vi "Eliminar ceros dentro de while o for V 2011.vi"() -> ()   [LabVIEW 2011]
panel:
  out "ELEMENTOS A UTILIZAR 0001  H":dbl[](array[numeric])
  out "reversed array 2":dbl[](array[numeric])
  out "reversed array":dbl[](array[numeric])
  out "appended array":dbl[](array[numeric])
  in  "stop":bool
  out "element":dbl
  in  "array":dbl[](array[numeric])=[3.0, 4.0, 0.0, 0.0, 2.0, 35.0, 0.0, 32.0, 0.0, 0.0, 12.0, 8.0, 6.0, 0.0, 2.0]
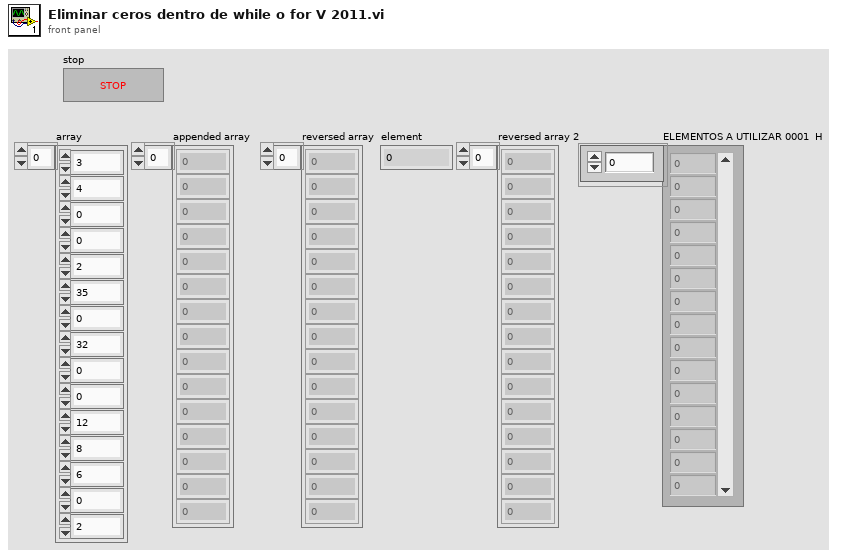
[diagram p1: front panel]
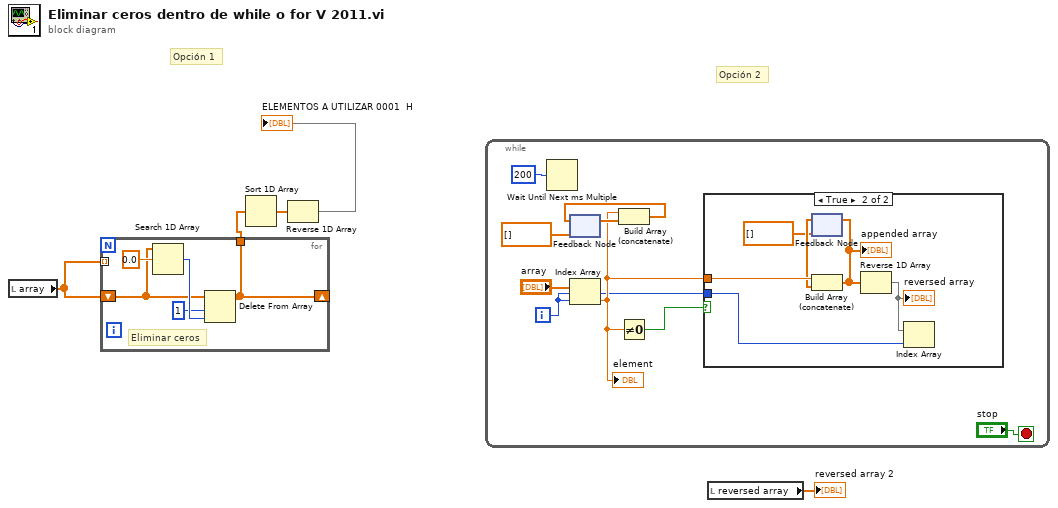
[diagram p0: block diagram]
diagram:
  # "Opción 2"
  # "Opción 1"
  n1 = local read "array"() -> (w1:dbl[])
  n2 = for {
    tunnel: [w7] -> w4
    shift-right: [w7] -> _
    shift-left: w1 -> [w6]
    tunnel: w1 -> [_] mode=indexing
    # "Eliminar ceros"
    n3 = Search 1D Array(1D array=w6, element=0.0) -> (index of element=w9:i32)  [unwired: 1 in]
    n4 = Delete From Array(array=w6, length=1, index=w9) -> (array with subset deleted=w7:dbl[])  [unwired: 1 out]
  }
  n5 = Sort 1D Array(array=w4) -> (sorted array=w3:dbl[])
  n6 = Reverse 1D Array(array=w3) -> (reversed array=→"ELEMENTOS A UTILIZAR 0001  H":dbl[])
  n7 = while {
    i -> [w12]
    stop <- "stop" stop-if-true
    n8 = Wait Until Next ms Multiple(millisecond multiple=u32 200) -> ()  [unwired: 1 out]
    n9 = feedback #1(dbl[] []) -> (w14:dbl[])
    n10 = Index Array(array="array", index=w12) -> (element=w13:dbl)
    "element" <- w13
    n11 = Build Array (concatenate)(w13, w14) -> (w16:dbl[])
    n12 = feedback-in #1(w16) -> ()
    n13 = Not Equal To 0?(x=w13) -> (x != 0?=w11:bool)
    n14 = case shown="True" w11 {
      tunnel: w13 -> [_ w25]
      tunnel: w12 -> [_ w20]
      frame False {
      }
      frame True {
        n15 = feedback #2(dbl[] []) -> (w24:dbl[])
        n16 = Build Array (concatenate)(w25, w24) -> (w22:dbl[])
        "appended array" <- w22
        n17 = feedback-in #2(w22) -> ()
        n18 = Reverse 1D Array(array=w22) -> (reversed array=w21:dbl[])
        "reversed array" <- w21
        n19 = Index Array(array=w21, index=w20) -> ()  [unwired: 1 out]
      }
    }
  }
  n20 = local read "reversed array"() -> (→"reversed array 2":dbl[])
